vi "FL_Check_TTL_firing_conditions.vi"(3 "Current segment' number (last value)":u32) -> (0 "TTL out N":u8, 1 "Fire TTL":bool)   [LabVIEW 2016]
uses:
  SW_Globals.vi
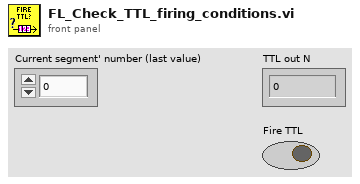
[diagram p1: front panel]
types:
  T1 = cluster{"Event type":u16, "Cond., s":sgl, "Stim., s":sgl, "Set/Clear":bool, "TTL out N":u16, "Stim. has been set":bool}[]
  T2 = cluster{"Event type":u16, "Cond., s":sgl, "Stim., s":sgl, "Set/Clear":bool, "TTL out N":u16, "Stim. has been set":bool}
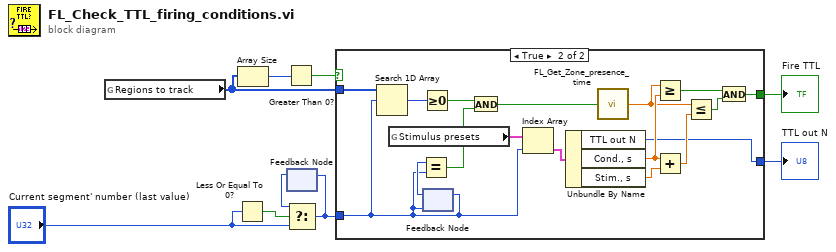
[diagram p0: block diagram]
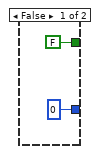
[diagram p2: hidden frame]
diagram:
  n1 = global read "SW_Globals.vi" "Regions to track"() -> (w3:u8[])
  n2 = Less Or Equal To 0?(x="Current segment' number (last value)") -> (x <= 0?=w6:bool)
  n3 = Array Size(array=w3) -> (size(s)=w1:i32)
  n4 = Greater Than 0?(x=w1) -> (x > 0?=w2:bool)
  n5 = feedback #1() -> (w5:u32)  [unwired: 1 in]
  n6 = Select(t=w5, s=w6, f="Current segment' number (last value)") -> (s? t:f=w4:u32)
  n7 = feedback-in #1(w4) -> ()
  n8 = case shown="True" w2 {
    tunnel: w4 -> [_ w23]
    tunnel: w3 -> [_ w26]
    tunnel: [FALSE w13] -> w8
    tunnel: [u16 0 w12] -> w9
    frame False {
    }
    frame True {
      n9 = Search 1D Array(1D array=w26, element=w23) -> (index of element=w27:i32)  [unwired: 1 in]
      n10 = global read "SW_Globals.vi" "Stimulus presets"() -> (w28:T1)
      n11 = Greater Or Equal To 0?(x=w27) -> (x >= 0?=w25:bool)
      n12 = feedback-in #2(w23) -> ()
      n13 = feedback #2(w23) -> (w24:u32)
      n14 = Equal?(x=w24, y=w23) -> (x = y?=w21:bool)
      n15 = And(x=w25, y=w21) -> (x .and. y?=w22:bool)
      n16 = Index Array(array=w28, index=w23) -> (element=w20:T2)
      n17 = Unbundle By Name(w20) -> ("TTL out N"=w12:u16, "Cond., s"=w19:sgl, "Stim., s"=w18:sgl)
      n18 = call "FL_Get_Zone_presence_time.vi"("Present in Zone"=w22) -> ("Zone presence time, s"=w14:dbl)
      n19 = Greater Or Equal?(x=w14, y=w19) -> (x >= y?=w15:bool)
      n20 = Add(x=w19, y=w18) -> (x+y=w17:sgl)
      n21 = Less Or Equal?(x=w14, y=w17) -> (x <= y?=w16:bool)
      n22 = And(x=w15, y=w16) -> (x .and. y?=w13:bool)
    }
  }
  "TTL out N" <- w9
  "Fire TTL" <- w8
